vi "dequeue_flexRIO.vi"(10 "make request?":bool, 11 "on-board buffer in":T1) -> (1 "output valid?":bool, 2 "data":u64, 3 "on-board buffer out":T1, 4 "iterations required for last retrieval":u32)   [LabVIEW 2010, in "OnBoardBuffer_flexRIO.lvlib"]
uses:
  OnBoardBuffer_flexRIO.lvlib
  <vilib>/rvi/DataTransferAndStorage/Container/XNode/niFpgaContainer.xnode
  OnBoardBuffer_flexRIO.ctl
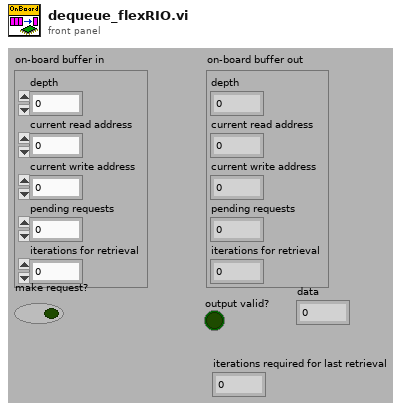
[diagram p1: front panel]
types:
  T1 = typedef "OnBoardBuffer_flexRIO.lvlib/OnBoardBuffer_flexRIO.ctl" = cluster{"depth":u32, "current read address":u32, "current write address":u32, "pending requests":u32, "iterations for retrieval":u32}
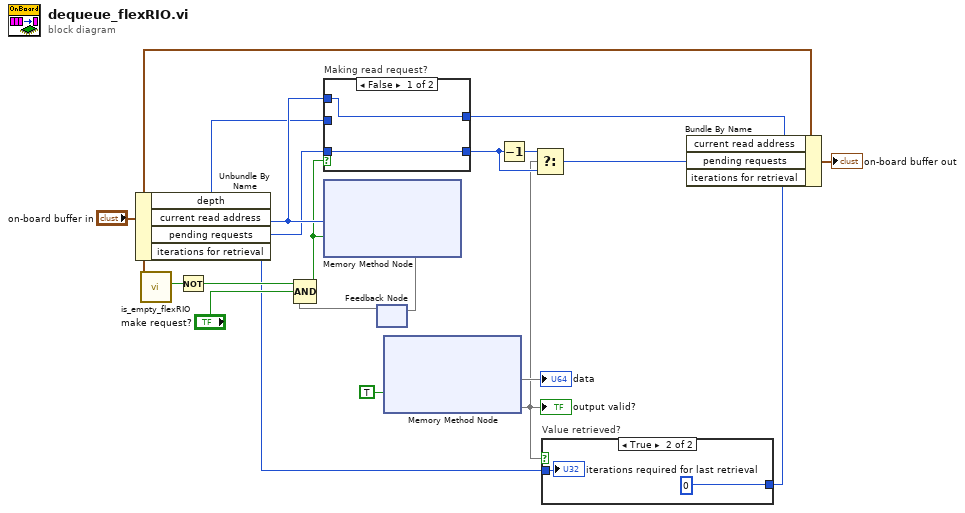
[diagram p0: block diagram]
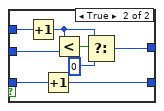
[diagram p2: hidden frame]
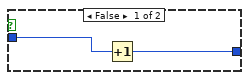
[diagram p3: hidden frame]
diagram:
  n1 = Unbundle By Name("on-board buffer in") -> ("depth"=w18:u32, "current read address"=w19:u32, "pending requests"=w12:u32, "iterations for retrieval"=w6:u32)
  n2 = call "is_empty_flexRIO.vi"("on-board buffer in"="on-board buffer in") -> ("is empty?"=w13:bool)  [unwired: 10 in]
  n3 = Not(x=w13) -> (.not. x?=w11:bool)
  n4 = feedback #1() -> (w3)  [unwired: 1 in]
  n5 = Compound Arithmetic op=AND(w11, "make request?", w3) -> (w1:bool)
  n6 = case "Making read request?" shown="False" w1 {
    tunnel: w19 -> [w21 w30]
    tunnel: w18 -> [_ w29]
    tunnel: [w21 w28] -> w17
    tunnel: w12 -> [w22 w27]
    tunnel: [w22 w26] -> w8
    frame False {
    }
    frame True {
      n7 = Increment(x=w30) -> (x+1=w25:u32)
      n8 = Increment(x=w27) -> (x+1=w26:u32)
      n9 = Less?(x=w25, y=w29) -> (x < y?=w23:bool)
      n10 = Select(t=w25, s=w23, f=u32 0) -> (s? t:f=w28:u32)
    }
  }
  n11 = xnode ("Memory Method Node")("Address"=w19, "Input Valid"=w1) -> ("Ready for Input"=w2)  [unwired: 1 in, 1 out]
  n12 = feedback-in #1(w2) -> ()
  n13 = xnode ("Memory Method Node")("Ready for Output"=TRUE) -> ("Data"=→"data", "Output Valid"=w5)  [unwired: 1 in, 1 out]
  "output valid?" <- w5
  n14 = Decrement(x=w8) -> (x-1=w9:u32)
  n15 = Select(t=w9, s=w5, f=w8) -> (s? t:f=w7:u32)
  n16 = case "Value retrieved?" shown="True" w5 {
    tunnel: w6 -> [w32 w34]
    tunnel: [w31 u32 0 ("t")] -> w4
    frame False {
      n17 = Increment(x=w32) -> (x+1=w31:u32)
    }
    frame True {
      "iterations required for last retrieval" <- w34
    }
  }
  n18 = Bundle By Name(cluster="on-board buffer in", "current read address"=w17, "pending requests"=w7, "iterations for retrieval"=w4) -> (→"on-board buffer out":T1)
